vi "20211008_02.vi"() -> ()   [LabVIEW 2019]
panel:
  out "Color Number":u32 format="%08d"
  in  "Color Box":u32(colorbox)
  in  "好感度 2":i32(slide) scale=0.0..4.0
  in  "好感度":dbl(slide) scale=0.0..4.0
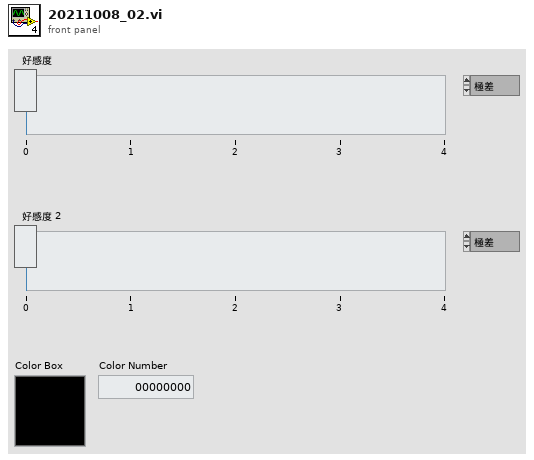
[diagram p1: front panel]
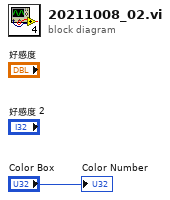
[diagram p0: block diagram]
diagram:
  "Color Number" <- "Color Box"
